vi "RT Task Monitor.vi"   [LabVIEW 2020]
doc: "This VI collects all the RT Task Status messages and periodically computes their statistics and reports them to the telemetry handler."
uses:
  Type Definitions/Real Time Task Status.ctl
  Type Definitions/Data Frame.ctl
  Type Definitions/Data Frame Header.ctl
  Type Definitions/Payload Class.ctl
  Type Definitions/Device.ctl
  Type Definitions/Enumerated Constants/Software Monitor.ctl
  Type Definitions/RTOSMonitor.ctl
  <vilib>/Analysis/baseanly.llb/Mean (DBL).vi
  <vilib>/Platform/TimedLoop/XDataNode/wakeup.ctl
  <vilib>/Platform/TimedLoop/XDataNode/XDNodeRunTimeDep.lvlib
  <vilib>/Platform/TimedLoop/XDataNode/nitl_modes.ctl
  <vilib>/Platform/TimedLoop/XDataNode/timing_clust.ctl
  <vilib>/platform/TimedLoop/XDataNode/XDataNode.xnode
  <vilib>/Analysis/NI_AALBase.lvlib
types:
  T1 = typedef "Real Time Task Status.ctl" = cluster{"Task Name":string, "Priority":i32, "Processor":i32, "Offset":i64, "Iteration Duration":i64, "Period":i64, "Finished Late":bool}
  T2 = typedef "Data Frame.ctl" = cluster{"Frame Header":T3, "Payload":string, "CRC":u32}
  T3 = typedef "Data Frame Header.ctl" = cluster{"Sync":u32, "Time":dbl, "Nanosecond Counter":i64, "Payload Class":T4, "Payload ID":u16, "Counter":i32, "Options":u32, "Source":T5, "Destination":T5}
  T4 = typedef "Payload Class.ctl" = enum16{"System State", "Parameters", "Metadata", "Software Monitor", "Data", "Commands"}
  T5 = typedef "Device.ctl" = enum32{"None", "Exec", "Aux1", "Aux2", "Aux3"}
  T6 = typedef "Software Monitor.ctl" = enum16{"Internet Connection Monitor", "CPU Monitor", "Archive Monitor", "Memory Monitor", "Queue Monitor", "RTOS Update", "RTOS Monitor"}
  T7 = typedef "RTOSMonitor.ctl" = cluster{"Task Name":string, "Priority":i32, "Processor":i32, "Offset":i64, "Min Duration":i64, "Mean Duration":i64, "Max Duration":i64, "Period":i64, "Late Iterations":i16, "Iteration Count":i32}
  T8 = typedef "XDNodeRunTimeDep.lvlib/timing_clust.ctl" = cluster{"Expected End [f-1]":u64, "Actual End [f-1]":u64, "Finished Late? [f-1]":bool, "Expected End [i-1]":u64, "Actual End [i-1]":u64, "Finished Late? [i-1]":bool, "Expected Start [i]":u64, "Actual Start [i]":u64, "Expected Start [f]":u64, "Actual Start [f]":u64, "Source Name":string, "Structure Name":string, "Period":i64, "Deadline":i64, "Offset":i64, "Start":i64, "Priority":i32, "Timeout":i32, "Mode":T9, "Wakeup Reason":T10, "Error":errorcluster, "Source Type":string, "Secondary Source Type":string, "Global End Time":u64, "Global Start Time":u64, "Frame Duration":u64, "Iteration Duration":u64, "Assigned CPU":i32, "I/O Scan Engine Mode":u32}
  T9 = typedef "XDNodeRunTimeDep.lvlib/nitl_modes.ctl" = enum32{"No Change", "Process missed periods, maintain original phase", "Discard missed periods, maintain original phase", "Process missed periods, ignore original phase", "Discard missed periods, ignore original phase"}
  T10 = typedef "XDNodeRunTimeDep.lvlib/wakeup.ctl" = enum32{"Normal", "Aborted", "Asynchronous wakeup", "Timing source error", "Timed loop error", "Timeout"}
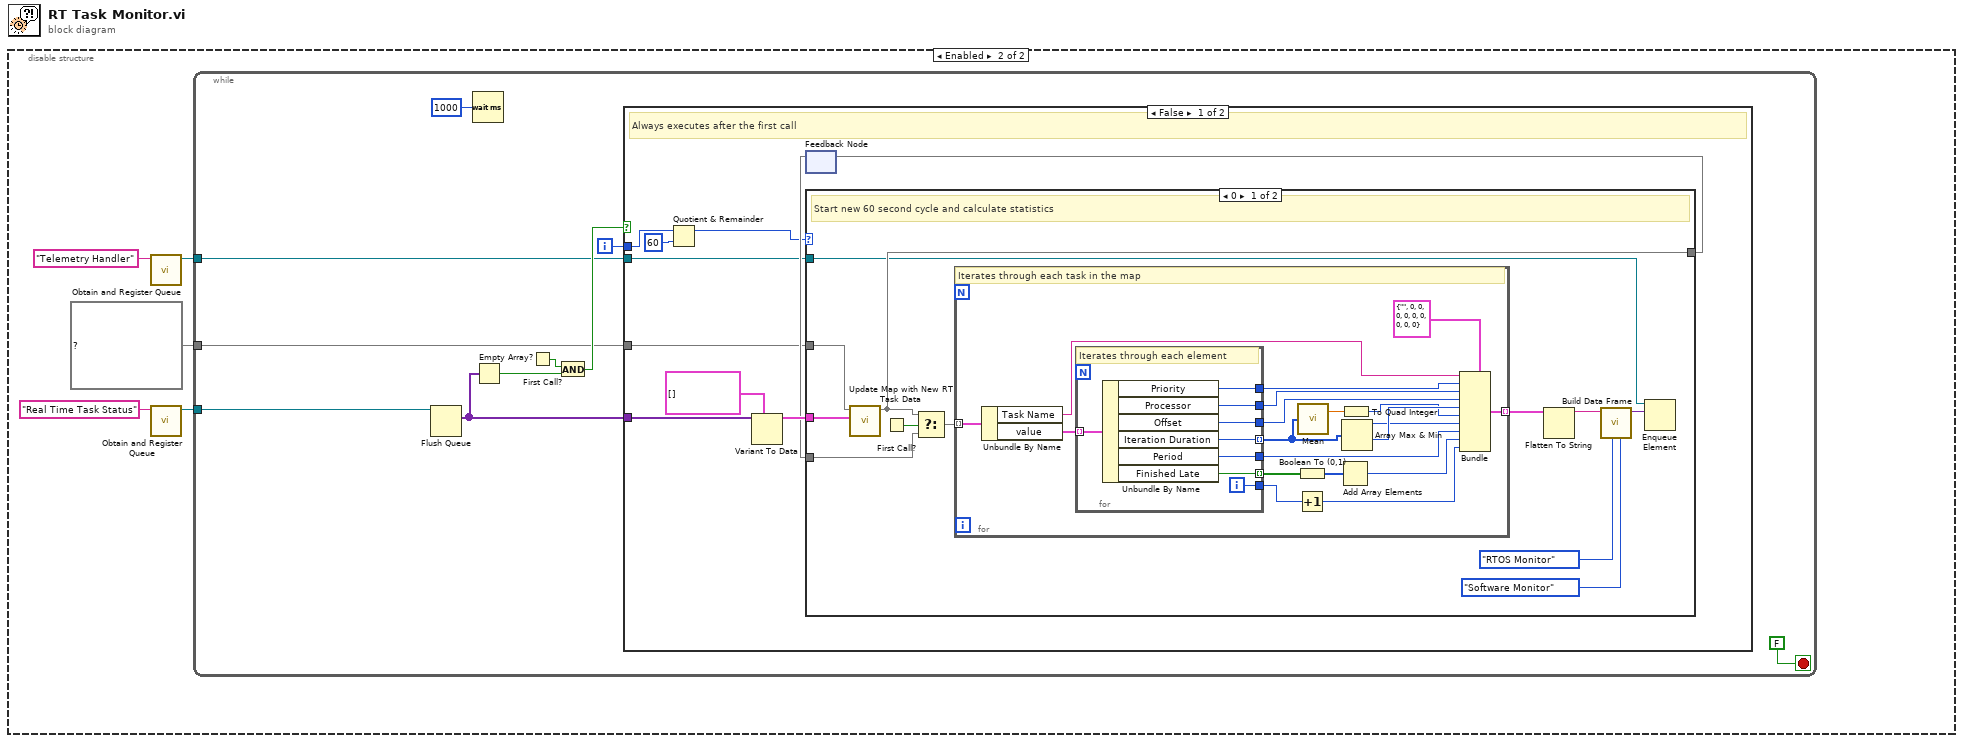
[diagram p0: block diagram]
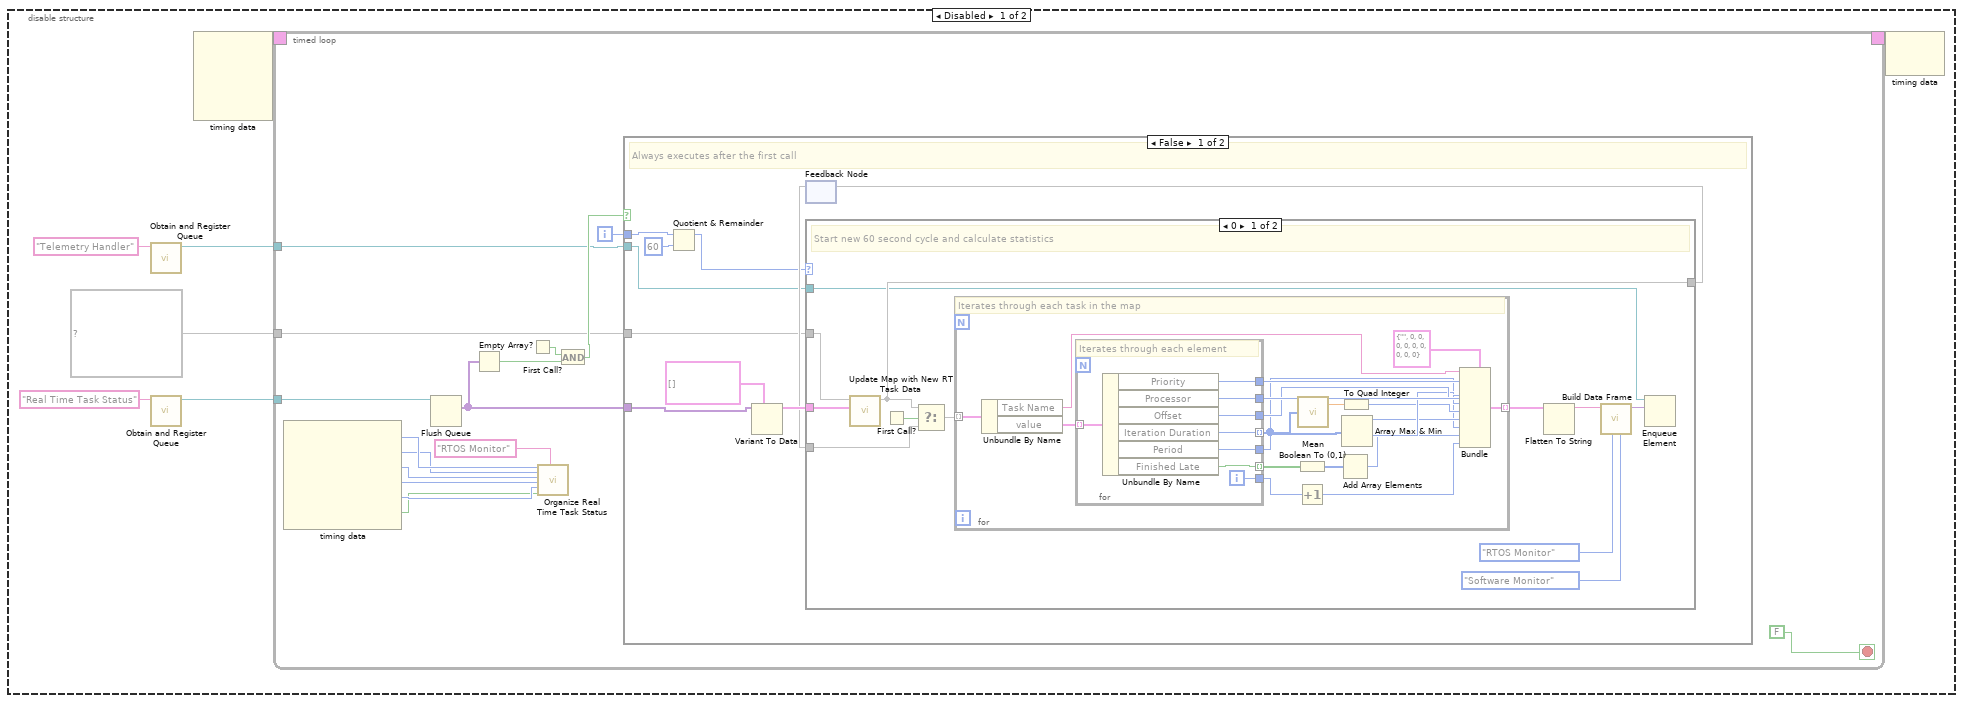
[diagram p2: hidden frame]
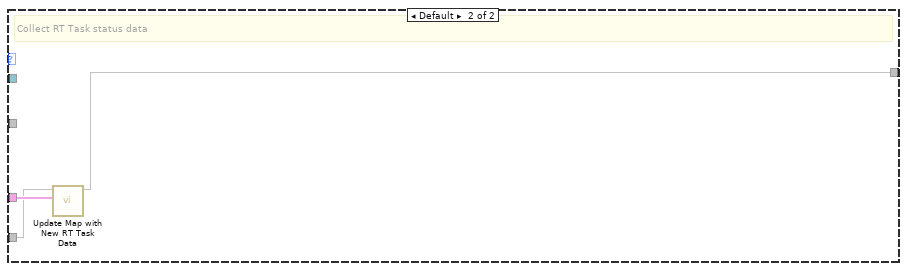
[diagram p3: hidden frame]
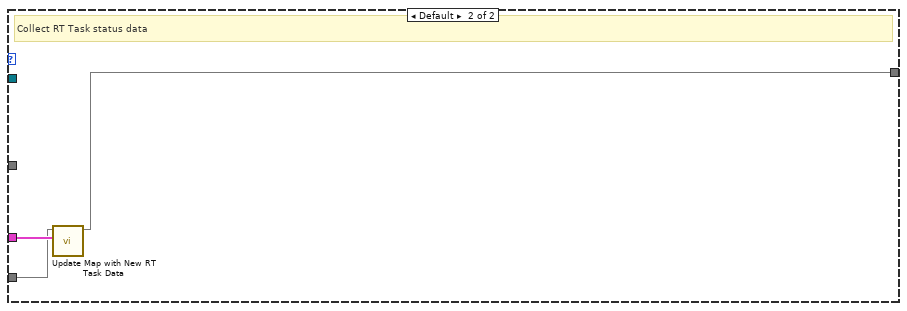
[diagram p5: hidden frame]
diagram:
  n1 = disable-structure shown="Enabled" {
    frame Disabled {
      n2 = call "Obtain and Register Queue.vi"("name (unnamed)"="Telemetry Handler") -> ("Queue Out"=w2:refnum<queue>)  [unwired: 7 in, 3 out]
      n3 = call "Obtain and Register Queue.vi"("name (unnamed)"="Real Time Task Status") -> ("Queue Out"=w5:refnum<queue>)  [unwired: 7 in, 3 out]
      n4 = node-c288() -> (w7:T8)  [unwired: 4 in]
      n5 = timed-loop {
        timing: w7 -> [_]
        timing-out: [_] -> w6
        tunnel: w5 -> [w15]
        tunnel: w2 -> [w9]
        tunnel: map{string, T1[]} {} ("map") -> [w8]
        i -> [w14]
        stop <- FALSE stop-if-true
        n6 = node-c288() -> (w21:i32, w20:i32, w19:i64, w18:i64, w17:i64, w16:bool)  [unwired: 1 in]
        n7 = Flush Queue(queue=w15) -> (remaining elements=w13:variant[])  [unwired: 1 in, 2 out]
        n8 = Empty Array?(array=w13) -> (empty?=w12:bool)
        n9 = First Call?() -> (First Call?: T/F=w11:bool)
        n10 = call "Organize Real Time Task Status.vi"("Priority"=w21, "Processor"=w20, "Offset"=w19, "Iteration Duration"=w18, "Period"=w17, "Finished Late? [i-1]"=w16, "Task Name"="RTOS Monitor") -> ()  [unwired: 12 in, 1 out]
        n11 = And(x=w11, y=w12) -> (x .and. y?=w10:bool)
        n12 = case shown="False" w10 {
          tunnel: w14 -> [w29 _]
          tunnel: w13 -> [w26 _]
          tunnel: w9 -> [w25 _]
          tunnel: w8 -> [w24 _]
          frame False {
            # "Always executes after the first call"
            n13 = Quotient & Remainder(x=w29, y=60) -> (x-y*floor(x/y)=w27:i32)  [unwired: 1 out]
            n14 = Variant To Data(type=T2[] [] ("Array"), Variant=w26) -> (data=w32:T2[])  [unwired: 1 in, 1 out]
            n15 = feedback #1() -> (w30:map{string, T1[]})  [unwired: 1 in]
            n16 = case shown="0" w27 {
              tunnel: w32 -> [w42 w75]
              tunnel: [w41 w74] -> w31
              tunnel: w30 -> [w44 w73]
              tunnel: w25 -> [w35 _]
              tunnel: w24 -> [w34 _]
              frame 0 {
                # "Start new 60 second cycle and calculate statistics"
                n17 = call "Update Map with New RT Task Data.vi"("RTOS Data"=w42, "RTOS Map In"=w34) -> ("RTOS Map Out"=w41:map{string, T1[]})  [unwired: 9 in]
                n18 = First Call?() -> (First Call?: T/F=w45:bool)
                n19 = Select(t=w41, s=w45, f=w44) -> (s? t:f=w43:map{string, T1[]})
                n20 = for {
                  tunnel: w43 -> [w61] mode=indexing
                  tunnel: [w46] -> w40 mode=indexing
                  # "Iterates through each task in the map"
                  n21 = Unbundle By Name(w61) -> ("Task Name"=w57:string, "value"=w64:T1[])
                  n22 = for {
                    tunnel: w64 -> [w72] mode=indexing
                    tunnel: [w71] -> w63 mode=indexing
                    tunnel: [w69] -> w60 mode=indexing
                    tunnel: [w70] -> w58
                    tunnel: [w68] -> w56
                    tunnel: [w67] -> w55
                    tunnel: [w66] -> w54
                    tunnel: [w65] -> w50
                    i -> [w70]
                    # "Iterates through each element"
                    n23 = Unbundle By Name(w72) -> ("Priority"=w68:i32, "Processor"=w67:i32, "Offset"=w66:i64, "Iteration Duration"=w71:i64, "Period"=w65:i64, "Finished Late"=w69:bool)
                  }
                  n24 = Boolean To (0,1)(Boolean=w60) -> (0, 1=w59:i16[])
                  n25 = Increment(x=w58) -> (x+1=w48:i32)
                  n26 = call-poly <vilib>:"Mean.vi"("X"=w63) -> ("mean"=w62:dbl)  [unwired: 1 out]
                  n27 = Add Array Elements(numeric array=w59) -> (sum=w49:i16)
                  n28 = To Quad Integer(1:w62) -> (0:w52:i64)
                  n29 = Array Max & Min(array=w63) -> (max value=w51:i64, min value=w53:i64)  [unwired: 2 out]
                  n30 = Bundle(cluster=T7 {"Task Name"="", "Priority"=0, "Processor"=0, "Offset"=0, "Min Duration"=0, "Mean Duration"=0, "Max Duration"=0, "Period"=0, "Late Iterations"=0, "Iteration Count"=0}, "Task Name"=w57, "Priority"=w56, "Processor"=w55, "Offset"=w54, "Min Duration"=w53, "Mean Duration"=w52, "Max Duration"=w51, "Period"=w50, "Late Iterations"=w49, "Iteration Count"=w48) -> (w46:T7)
                }
                n31 = Flatten To String(anything=w40) -> (data string=w37:string)  [unwired: 3 in, 2 out]
                n32 = call "Build Data Frame.vi"("Payload Class (Data)"=Payload_Class."Software Monitor", "Payload ID (0)"=Software_Monitor."RTOS Monitor", "Payload (Empty String)"=w37) -> ("Frame"=w36:variant)  [unwired: 7 in, 1 out]
                n33 = Enqueue Element(queue=w35, element=w36) -> ()  [unwired: 2 in, 3 out]
              }
              frame Default {
                # "Collect RT Task status data"
                n34 = call "Update Map with New RT Task Data.vi"("RTOS Data"=w75, "RTOS Map In"=w73) -> ("RTOS Map Out"=w74:map{string, T1[]})  [unwired: 9 in]
              }
            }
            n35 = feedback-in #1(w31) -> ()
          }
          frame True {
            # "Makes sure loop does not execute on first call if there are no elements in the RT Task array"
          }
        }
      }
      n36 = node-c288(w6) -> ()  [unwired: 1 out]
    }
    frame Enabled {
      n37 = call "Obtain and Register Queue.vi"("name (unnamed)"="Telemetry Handler") -> ("Queue Out"=w87:refnum<queue>)  [unwired: 7 in, 3 out]
      n38 = call "Obtain and Register Queue.vi"("name (unnamed)"="Real Time Task Status") -> ("Queue Out"=w90:refnum<queue>)  [unwired: 7 in, 3 out]
      n39 = while {
        tunnel: w90 -> [w99]
        tunnel: w87 -> [w93]
        tunnel: map{string, T1[]} {} ("map") -> [w91]
        i -> [w98]
        stop <- FALSE stop-if-true
        n40 = Flush Queue(queue=w99) -> (remaining elements=w97:variant[])  [unwired: 1 in, 2 out]
        n41 = Wait (ms)(milliseconds to wait=u32 1000) -> ()  [unwired: 1 out]
        n42 = Empty Array?(array=w97) -> (empty?=w96:bool)
        n43 = First Call?() -> (First Call?: T/F=w95:bool)
        n44 = And(x=w95, y=w96) -> (x .and. y?=w94:bool)
        n45 = case shown="False" w94 {
          tunnel: w98 -> [w106 _]
          tunnel: w97 -> [w103 _]
          tunnel: w93 -> [w102 _]
          tunnel: w91 -> [w101 _]
          frame False {
            # "Always executes after the first call"
            n46 = Quotient & Remainder(x=w106, y=60) -> (x-y*floor(x/y)=w104:i32)  [unwired: 1 out]
            n47 = Variant To Data(type=T2[] [] ("Array"), Variant=w103) -> (data=w109:T2[])  [unwired: 1 in, 1 out]
            n48 = feedback #2() -> (w107:map{string, T1[]})  [unwired: 1 in]
            n49 = case shown="0" w104 {
              tunnel: w109 -> [w119 w152]
              tunnel: [w118 w151] -> w108
              tunnel: w107 -> [w121 w150]
              tunnel: w102 -> [w112 _]
              tunnel: w101 -> [w111 _]
              frame 0 {
                # "Start new 60 second cycle and calculate statistics"
                n50 = call "Update Map with New RT Task Data.vi"("RTOS Data"=w119, "RTOS Map In"=w111) -> ("RTOS Map Out"=w118:map{string, T1[]})  [unwired: 9 in]
                n51 = First Call?() -> (First Call?: T/F=w122:bool)
                n52 = Select(t=w118, s=w122, f=w121) -> (s? t:f=w120:map{string, T1[]})
                n53 = for {
                  tunnel: w120 -> [w138] mode=indexing
                  tunnel: [w123] -> w117 mode=indexing
                  # "Iterates through each task in the map"
                  n54 = Unbundle By Name(w138) -> ("Task Name"=w134:string, "value"=w141:T1[])
                  n55 = for {
                    tunnel: w141 -> [w149] mode=indexing
                    tunnel: [w148] -> w140 mode=indexing
                    tunnel: [w146] -> w137 mode=indexing
                    tunnel: [w147] -> w135
                    tunnel: [w145] -> w133
                    tunnel: [w144] -> w132
                    tunnel: [w143] -> w131
                    tunnel: [w142] -> w127
                    i -> [w147]
                    # "Iterates through each element"
                    n56 = Unbundle By Name(w149) -> ("Priority"=w145:i32, "Processor"=w144:i32, "Offset"=w143:i64, "Iteration Duration"=w148:i64, "Period"=w142:i64, "Finished Late"=w146:bool)
                  }
                  n57 = Boolean To (0,1)(Boolean=w137) -> (0, 1=w136:i16[])
                  n58 = Increment(x=w135) -> (x+1=w125:i32)
                  n59 = call-poly <vilib>:"Mean.vi"("X"=w140) -> ("mean"=w139:dbl)  [unwired: 1 out]
                  n60 = Add Array Elements(numeric array=w136) -> (sum=w126:i16)
                  n61 = To Quad Integer(1:w139) -> (0:w129:i64)
                  n62 = Array Max & Min(array=w140) -> (max value=w128:i64, min value=w130:i64)  [unwired: 2 out]
                  n63 = Bundle(cluster=T7 {"Task Name"="", "Priority"=0, "Processor"=0, "Offset"=0, "Min Duration"=0, "Mean Duration"=0, "Max Duration"=0, "Period"=0, "Late Iterations"=0, "Iteration Count"=0}, "Task Name"=w134, "Priority"=w133, "Processor"=w132, "Offset"=w131, "Min Duration"=w130, "Mean Duration"=w129, "Max Duration"=w128, "Period"=w127, "Late Iterations"=w126, "Iteration Count"=w125) -> (w123:T7)
                }
                n64 = Flatten To String(anything=w117) -> (data string=w114:string)  [unwired: 3 in, 2 out]
                n65 = call "Build Data Frame.vi"("Payload Class (Data)"=Payload_Class."Software Monitor", "Payload ID (0)"=Software_Monitor."RTOS Monitor", "Payload (Empty String)"=w114) -> ("Frame"=w113:variant)  [unwired: 7 in, 1 out]
                n66 = Enqueue Element(queue=w112, element=w113) -> ()  [unwired: 2 in, 3 out]
              }
              frame Default {
                # "Collect RT Task status data"
                n67 = call "Update Map with New RT Task Data.vi"("RTOS Data"=w152, "RTOS Map In"=w150) -> ("RTOS Map Out"=w151:map{string, T1[]})  [unwired: 9 in]
              }
            }
            n68 = feedback-in #2(w108) -> ()
          }
          frame True {
            # "Makes sure loop does not execute on first call if there are no elements in the RT Task array"
          }
        }
      }
    }
  }
